vi "testCreateNotifier.vi"(8 "error in (no error)":errorcluster) -> (0 "error out":errorcluster)   [LabVIEW 2018]
doc: "Test the createNotifier.vi."
uses:
  src/TcpServerBase/TcpServerBase.lvclass
  src/TcpServerBase/TcpServerBase.lvclass/TcpServerBase.ctl
  <vilib>/addons/_JKI Toolkits/Caraya/classes/Assert/Assert Equal Type_Variant.vi
  <vilib>/addons/_JKI Toolkits/Caraya/classes/Test/Test.lvclass
  <vilib>/addons/_JKI Toolkits/Caraya/classes/Assert/Assert.lvclass
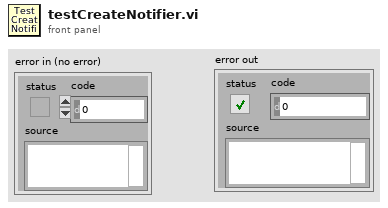
[diagram p1: front panel]
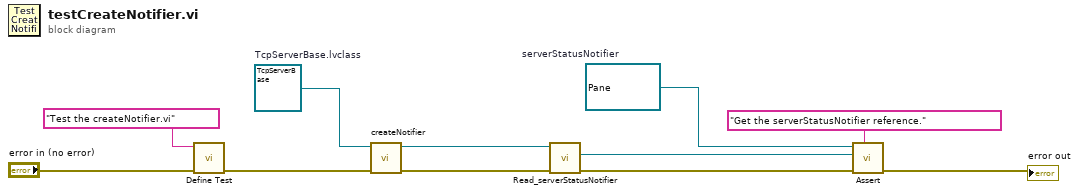
[diagram p0: block diagram]
diagram:
  w2 = refnum<notifier> refnum  # serverStatusNotifier
  w7 = refnum<class "TcpServerBase.lvclass"> refnum  # TcpServerBase.lvclass
  n1 = call <vilib>:"Define Test.vi"("error in (no error)"="error in (no error)", "Label (VI Title)"="Test the createNotifier.vi") -> ("error out"=w6:errorcluster)  [unwired: 9 in]
  n2 = call "createNotifier.vi"("error in (no error)"=w6, "tcpServerBase in"=w7) -> ("error out"=w4:errorcluster, "tcpServerBase out"=w5:refnum<class "TcpServerBase.lvclass">)  [unwired: 8 in]
  n3 = call "Read_serverStatusNotifier.vi"("error in (no error)"=w4, "TcpServerBase in"=w5) -> ("error out"=w3:errorcluster, "serverStatusNotifier"=w1:refnum<notifier>)  [unwired: 7 in, 1 out]
  n4 = call-poly <vilib>:"Assert.vi"("Label"="Get the serverStatusNotifier reference.", "error in (no error)"=w3, "Y"=w1, "X"=w2) -> ("error out"=→"error out":errorcluster)  [unwired: 7 in]
